vi "Vision Processing.vi"(4 "error in (no error)":errorcluster, 7 "Image Size":T3=enum."320x240") -> ()   [LabVIEW 2016]
doc: "This VI runs in parallel to other tasks. It gets images from the camera, processes them for color or shape and use that information to affect robot behavior."
uses:
  <vilib>/Rock Robotics/WPI/Camera/WPI_CameraImageSize.ctl
  <vilib>/Rock Robotics/WPI/Camera/WPI_CameraWhite Balance Values.ctl
  <vilib>/Rock Robotics/WPI/Camera/WPI_CameraExposure Values.ctl
  <vilib>/Rock Robotics/WPI/Camera/WPI_CameraFrameRate.ctl
  Robot Global Data.vi
panel:
  out "Target Data":T1
  out "Delay":u32
  out "Tiltedness":dbl
  out "Camera Image":T2(plugin-control)
  in  "Vision Target":enum16{"Pegs", "Gears"}(ring)
  out "Binary Image":T2(plugin-control)
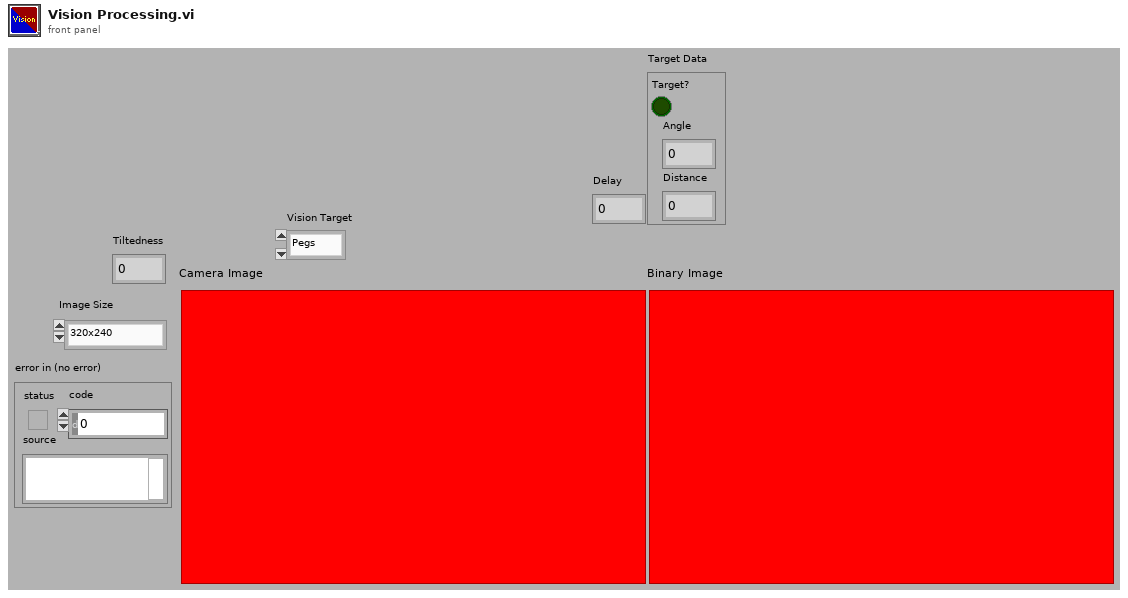
[diagram p1: front panel]
types:
  T1 = cluster{"Target?":bool, "Angle":dbl, "Distance":dbl}
  T2 = typedef "IMAQ Image.ctl" = refnum<image>
  T3 = typedef "WPI_CameraImageSize.ctl" = enum16{"640x480", "320x240", "160x120", "Custom"}
  T4 = typedef "WPI_CameraFrameRate.ctl" = u32
  T5 = typedef "WPI_CameraExposure Values.ctl" = enum16{"Auto", "Flicker-free 50 Hz", "Flicker-free 60 Hz", "Hold current", "Custom"}
  T6 = typedef "WPI_CameraWhite Balance Values.ctl" = enum16{"Auto", "Fixed indoor", "Fixed outdoor 1", "Fixed outdoor 2", "Fixed fluorescent 1", "Fixed fluorescent 2", "Hold current", "Custom"}
  T7 = typedef "Image Type" = u32
  T8 = typedef "WPI_CameraDevRef.ctl" = cluster{"Camera Address":string, "CameraStatus":errorcluster}
  T9 = cluster{"Target?":bool, "PegAngle":dbl, "Distance":dbl}
  T10 = typedef "WPI_EncoderDevRef.ctl" = cluster{"DevStatus":errorcluster, "EncoderIndex":T11, "CounterIndex":T12, "DistancePerCount":dbl, "Decoding Type":T13}
  T11 = typedef "FPGA_EncoderIdx.ctl" = enum8{"Enc 0", "Enc 1", "Enc 2", "Enc 3", "Enc 4", "Enc 5", "Enc 6", "Enc 7", "Invalid"}
  T12 = typedef "FPGA_CounterCtrSystemIndex.ctl" = enum8{"Ctr 0", "Ctr 1", "Ctr 2", "Ctr 3", "Ctr 4", "Ctr 5", "Ctr 6", "Ctr 7", "Invalid"}
  T13 = typedef "WPI_EncoderType.ctl" = enum16{"1x", "2x", "4x"}
  T14 = cluster{"Left":cluster{"L":dbl, "T":dbl, "R":dbl, "B":dbl, "X":dbl, "Y":dbl}, "Right":cluster{"L":dbl, "T":dbl, "R":dbl, "B":dbl, "X":dbl, "Y":dbl}}
  T15 = cluster{"Rectangle":cluster{"L":dbl, "T":dbl, "R":dbl, "B":dbl}, "Center":cluster{"X":dbl, "Y":dbl}}
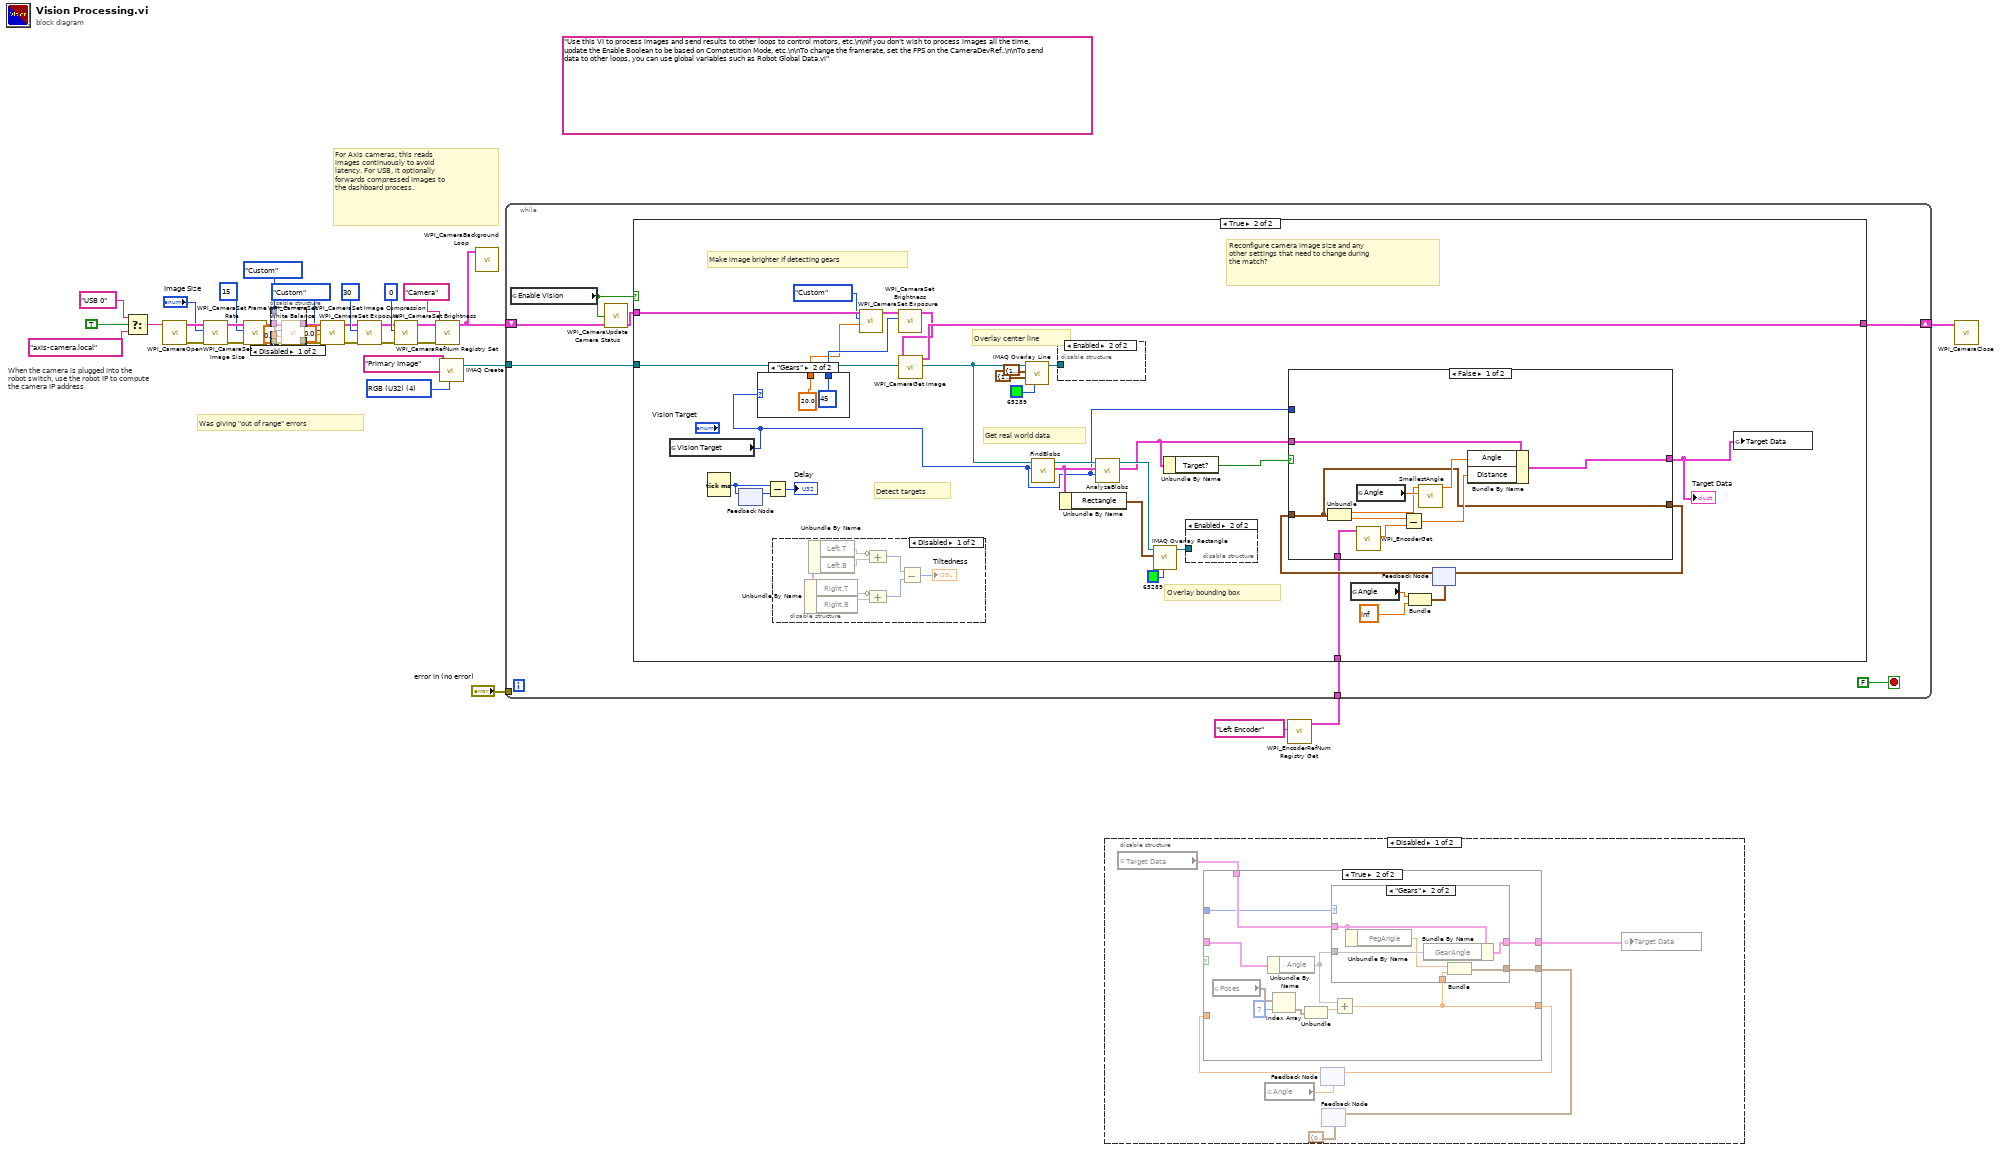
[diagram p0: block diagram]
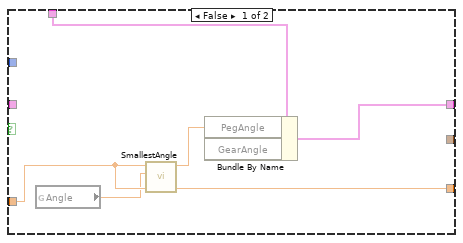
[diagram p2: hidden frame]
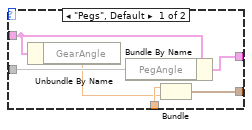
[diagram p3: hidden frame]
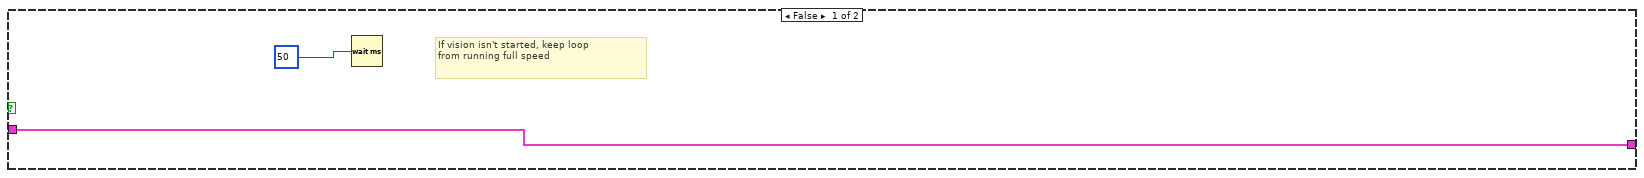
[diagram p6: hidden frame]
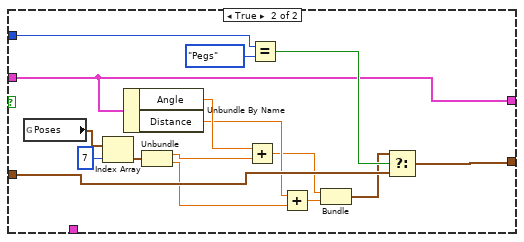
[diagram p7: hidden frame]
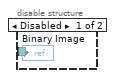
[diagram p9: hidden frame]
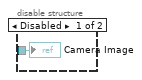
[diagram p10: hidden frame]
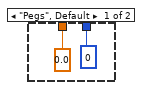
[diagram p11: hidden frame]
diagram:
  (unwired) "Use this VI to process images and send results to other loops to control motors, etc.\n\nIf you don't wish to process images all the time, update the Enable Boolean to be based on Comptetition Mode, etc.\n\nTo change the framerate, set the FPS on the CameraDevRef..\n\nTo send data to other loops, you can use global variables such as Robot Global Data.vi"
  w35 = T7 4 items=["Grayscale (U8)", "Grayscale (I16)", "Grayscale (SGL)", "Complex (CSG)", "RGB (U32)", "HSL (U32)", "RGB (U64)"] ("Image Type")
  # "Was giving \"out of range\" errors"
  # "When the camera is plugged into the\nrobot switch, use the robot IP to compute\nthe camera IP address"
  # "For Axis cameras, this reads\nimages continuously to avoid\nlatency. For USB, it optionally\nforwards compressed images to\nthe dashboard process."
  n1 = Select(t="USB 0" ("format string"), s=TRUE ("dot notation? (F)"), f="axis-camera.local" ("format string")) -> (s? t:f=w6:string)
  n2 = call <vilib>:"WPI_CameraOpen.vi"("Camera Address"=w6) -> ("error out"=w23:errorcluster, "CameraDevRef"=w24:T8)  [unwired: 1 in, 8 out]
  n3 = call <vilib>:"WPI_CameraSet Image Size.vi"("error in (no error)"=w23, "Image Size"="Image Size", "CameraDevRef"=w24) -> ("error out"=w22:errorcluster, "CameraDevRef Out"=w25:T8)  [unwired: 1 in, 6 out]
  n4 = call <vilib>:"WPI_CameraSet Frame Rate.vi"("error in (no error)"=w22, "Frame Rate (fps)"=T4 15, "CameraDevRef"=w25) -> ("error out"=w21:errorcluster, "CameraDevRef Out"=w27:T8)  [unwired: 7 out]
  n5 = disable-structure shown="Disabled" {
    disable-tunnel: w27 -> [w41 w43]
    disable-tunnel: [w40 w43] -> w26
    disable-tunnel: w21 -> [w39 w42]
    disable-tunnel: [w38 w42] -> w20
    disable-tunnel: WPI_CameraWhite_Balance_Values."Custom" ("White Balance") -> [w37 _]
    disable-tunnel: 0.0 ("Color Temp (K)") -> [w36 _]
    frame Disabled {
      n6 = call <vilib>:"WPI_CameraSet White Balance.vi"("error in (no error)"=w39, "Color Temp (K)"=w36, "White Balance"=w37, "CameraDevRef"=w41) -> ("error out"=w38:errorcluster, "CameraDevRef Out"=w40:T8)  [unwired: 6 out]
    }
    frame Enabled {
    }
  }
  n7 = call <vilib>:"WPI_CameraSet Exposure.vi"("error in (no error)"=w20, "Exposure (%)"=0.0, "Exposure"=WPI_CameraExposure_Values."Custom", "CameraDevRef"=w26) -> ("error out"=w19:errorcluster, "CameraDevRef Out"=w29:T8)  [unwired: 6 out]
  n8 = call <vilib>:"WPI_CameraSet Image Compression.vi"("error in (no error)"=w19, "Compression"=30, "CameraDevRef"=w29) -> ("error out"=w18:errorcluster, "CameraDevRef Out"=w28:T8)  [unwired: 7 out]
  n9 = call <vilib>:"WPI_CameraSet Brightness.vi"("error in (no error)"=w18, "Brightness"=0, "CameraDevRef"=w28) -> ("error out"=w16:errorcluster, "CameraDevRef Out"=w17:T8)  [unwired: 7 out]
  n10 = call <vilib>:"WPI_CameraRefNum Registry Set.vi"("error in (no error)"=w16, "refnum name"="Camera", "CameraDevRef"=w17) -> ("CameraDevRef"=w12:T8)  [unwired: 1 in, 7 out]
  n11 = call "IMAQ Create"("Image Name"="Primary Image", "Image Type"=w35) -> ("New Image"=w33:T2)  [unwired: 2 in, 2 out]
  n12 = call <vilib>:"WPI_CameraBackground Loop.vi"("CameraDevRef"=w12) -> ()  [unwired: 11 in]
  n13 = disable-structure shown="Disabled" {
    frame Disabled {
      n14 = global read "Robot Global Data.vi" "Target Data"() -> (w47:T9)
      n15 = global read "Robot Global Data.vi" "Angle"() -> (w48:dbl)
      n16 = feedback #1(w48) -> (w50:dbl)
      n17 = case shown="True" {
        selector: _ -> [_ _]
        tunnel: [w55 w59] -> w46
        tunnel: _ -> [_ w60]
        tunnel: [w54 w56] -> w49
        tunnel: w50 -> [w54 _]
        tunnel: w47 -> [w51 w62]
        tunnel: _ -> [_ w58]
        tunnel: [_ w57] -> w44
        frame False {
          n18 = global read "Robot Global Data.vi" "Angle"() -> (w53:dbl)
          n19 = call "SmallestAngle.vi"("Angle 2"=w53, "Angle 1"=w54) -> ("Smallest Difference"=w52:dbl)  [unwired: 9 in]
          n20 = Bundle By Name(cluster=w51, "PegAngle"=w52) -> (w55:T9)  [unwired: 1 in]
        }
        frame True {
          n21 = global read "Robot Global Data.vi" "Poses"() -> (w66:cluster{"theta":dbl, "distance":dbl}[])
          n22 = Unbundle By Name(w60) -> ("Angle"=w61)
          n23 = Index Array(array=w66, index=7) -> (element=w64:cluster{"theta":dbl, "distance":dbl})
          n24 = Unbundle(w64) -> ("theta"=w63:dbl)  [unwired: 1 out]
          n25 = Add(x=w61, y=w63) -> (x+y=w56:dbl)
          n26 = case shown="\"Gears\"" w58 {
            tunnel: w62 -> [w68 w74]
            tunnel: w61 -> [w71 w78]
            tunnel: [w72 w77] -> w59
            tunnel: [w70 w75] -> w57
            tunnel: w56 -> [w69 w76]
            frame "Pegs", Default {
              n27 = Unbundle By Name(w68) -> ("GearAngle"=w67:dbl)
              n28 = Bundle By Name(cluster=w68, "PegAngle"=w71) -> (w72:T9)
              n29 = Bundle(w69, "GearAngle"=w67) -> (w70:cluster{dbl, "GearAngle":dbl})  [unwired: 1 in]
            }
            frame "Gears" {
              n30 = Unbundle By Name(w74) -> ("PegAngle"=w73:dbl)
              n31 = Bundle By Name(cluster=w74, "GearAngle"=w78) -> (w77:T9)
              n32 = Bundle("PegAngle"=w73, w76) -> (w75:cluster{"PegAngle":dbl, dbl})  [unwired: 1 in]
            }
          }
        }
      }
      n33 = feedback-in #1(w49) -> ()
      n34 = feedback #2(cluster{"PegAngle":dbl, "GearAngle":dbl} {"PegAngle"=0.0, "GearAngle"=0.0} ("Target Data")) -> ()  [unwired: 1 in]
      n35 = feedback-in #2(w44) -> ()
      n36 = global write "Robot Global Data.vi" "Target Data"(w46) -> ()
    }
    frame Enabled {
    }
  }
  n37 = call <vilib>:"WPI_EncoderRefNum Registry Get.vi"("refnum name"="Left Encoder") -> ("EncoderDevRef"=w1:T10)  [unwired: 9 in, 1 out]
  n38 = while {
    shift-right: [w84] -> w10
    shift-left: w12 -> [w82]
    tunnel: w33 -> [w83]
    tunnel: "error in (no error)" -> [_]
    tunnel: w1 -> [w79]
    stop <- FALSE stop-if-true
    n39 = global read "Robot Global Data.vi" "Enable Vision"() -> (w80:bool)
    n40 = call <vilib>:"WPI_CameraUpdate Camera Status.vi"("CameraDevRef In"=w82, "Enable Vision"=w80) -> ("CameraDevRef Out"=w81:T8)  [unwired: 3 in]
    n41 = case shown="True" w80 {
      tunnel: w83 -> [_ w119]
      tunnel: [w87 w118] -> w84
      tunnel: w81 -> [w87 w107]
      tunnel: w79 -> [_ w91]
      frame False {
        # "If vision isn't started, keep loop\nfrom running full speed"
        n42 = Wait (ms)(milliseconds to wait=u32 50) -> ()  [unwired: 1 out]
      }
      frame True {
        # "Get real world data"
        # "Detect targets"
        # "Make image brighter if detecting gears"
        # "Overlay center line"
        # "Overlay bounding box"
        # "Reconfigure camera image size and any\nother settings that need to change during\nthe match?"
        n43 = global read "Robot Global Data.vi" "Vision Target"() -> (w93:enum16{"Pegs", "Gears"})
        n44 = Tick Count (ms)() -> (millisecond timer value=w102:u32)
        n45 = feedback-in #3(w102) -> ()
        n46 = feedback #3() -> (w103:u32)  [unwired: 1 in]
        n47 = case shown="\"Gears\"" w93 {
          tunnel: [0 ("Brightness") 45 ("Brightness")] -> w105
          tunnel: [0.0 ("Color Temp (K)") 20.0 ("Color Temp (K)")] -> w104
          frame "Pegs", Default {
          }
          frame "Gears" {
          }
        }
        n48 = Subtract(x=w102, y=w103) -> (x-y=→"Delay":u32)
        n49 = disable-structure shown="Disabled" {
          frame Disabled {
            n50 = Unbundle By Name() -> (w153:T14, "Left.T"=w152, "Left.B"=w151)
            n51 = Unbundle By Name(w153) -> ("Right.T"=w150, "Right.B"=w149)
            n52 = Compound Arithmetic op=ADD(invert w152, w151) -> (w148:i32)
            n53 = Compound Arithmetic op=ADD(invert w150, w149) -> (w147:i32)
            n54 = Subtract(x=w148, y=w147) -> (x-y=→"Tiltedness":i32)
          }
          frame Enabled {
          }
        }
        n55 = call <vilib>:"WPI_CameraSet Exposure.vi"("Exposure (%)"=w104, "Exposure"=WPI_CameraExposure_Values."Custom", "CameraDevRef"=w107) -> ("CameraDevRef Out"=w100:T8)  [unwired: 1 in, 7 out]
        n56 = call <vilib>:"WPI_CameraSet Brightness.vi"("Brightness"=w105, "CameraDevRef"=w100) -> ("CameraDevRef Out"=w106:T8)  [unwired: 1 in, 8 out]
        n57 = call <vilib>:"WPI_CameraGet Image.vi"("Image"=w119, "CameraDevRef"=w106) -> ("Image Out"=w109:T2, "CameraDevRef Out"=w118:T8)  [unwired: 1 in, 7 out]
        n58 = call "IMAQ Overlay Line"("Color"=u32 65289, "End Point"=cluster{"X":i32, "Y":i32} {"X"=160, "Y"=240}, "Start Point"=cluster{"X":i32, "Y":i32} {"X"=160, "Y"=0}, "Image"=w109) -> ("Image Out"=w108:T2)  [unwired: 6 in, 1 out]
        n59 = call "FindBlobs.vi"("Vision Target"=w93, "Image In"=w109) -> ("Blob Data"=w114:T15, "Image Out"=w98:T2)  [unwired: 8 in]
        n60 = disable-structure shown="Enabled" {
          disable-tunnel: w108 -> [w155 _]
          frame Disabled {
            "Camera Image" <- w155
          }
          frame Enabled {
          }
        }
        n61 = Unbundle By Name(w114) -> ("Rectangle"=w113:cluster{"L":dbl, "T":dbl, "R":dbl, "B":dbl})
        n62 = call "AnalyzeBlobs.vi"("Vision Target"=w93, "Blob Data"=w114, "Image In"=w98) -> ("Target Data"=w96:T1, "Image Out"=w115:T2)  [unwired: 7 in]
        n63 = call "IMAQ Overlay Rectangle"("Color"=u32 65289, "Rectangle"=w113, "Image"=w115) -> ("Image Out"=w116:T2)  [unwired: 7 in, 1 out]
        n64 = Unbundle By Name(w96) -> ("Target?"=w97:bool)
        n65 = disable-structure shown="Enabled" {
          disable-tunnel: w116 -> [w154 _]
          frame Disabled {
            "Binary Image" <- w154
          }
          frame Enabled {
          }
        }
        n66 = global read "Robot Global Data.vi" "Angle"() -> (w90:dbl)
        n67 = Bundle("Angle"=w90, "Distance"=inf) -> (w89:cluster{"Angle":dbl, "Distance":dbl})  [unwired: 1 in]
        n68 = feedback #4(w89) -> (w95:cluster{"Angle":dbl, "Distance":dbl})
        n69 = case shown="False" w97 {
          tunnel: w96 -> [w127 w138]
          tunnel: [w120 w133] -> w94
          tunnel: w95 -> [w120 w139]
          tunnel: w93 -> [_ w142]
          tunnel: [w126 w138] -> w92
          tunnel: w91 -> [w124 _]
          frame False {
            n70 = Unbundle(w120) -> ("Angle"=w125:dbl, "Distance"=w123:dbl)
            n71 = global read "Robot Global Data.vi" "Angle"() -> (w129:dbl)
            n72 = call <vilib>:"WPI_EncoderGet.vi"("EncoderDevRef"=w124) -> ("Distance"=w122:dbl)  [unwired: 5 in, 5 out]
            n73 = Subtract(x=w123, y=w122) -> (x-y=w121:dbl)
            n74 = call "SmallestAngle.vi"("Angle 2"=w129, "Angle 1"=w125) -> ("Smallest Difference"=w128:dbl)  [unwired: 9 in]
            n75 = Bundle By Name(cluster=w127, "Angle"=w128, "Distance"=w121) -> (w126:T1)
          }
          frame True {
            n76 = global read "Robot Global Data.vi" "Poses"() -> (w145:cluster{"theta":dbl, "distance":dbl}[])
            n77 = Index Array(array=w145, index=7) -> (element=w132:cluster{"theta":dbl, "distance":dbl})
            n78 = Unbundle By Name(w138) -> ("Angle"=w143:dbl, "Distance"=w137:dbl)
            n79 = Unbundle(w132) -> ("theta"=w131:dbl, "distance"=w130:dbl)
            n80 = Add(x=w143, y=w131) -> (x+y=w135:dbl)
            n81 = Equal?(x=w142, y=enum16{"Pegs", "Gears"}."Pegs") -> (x = y?=w140:bool)
            n82 = Add(x=w137, y=w130) -> (x+y=w136:dbl)
            n83 = Bundle(w135, w136) -> (w134:cluster{dbl, dbl})  [unwired: 1 in]
            n84 = Select(t=w134, s=w140, f=w139) -> (s? t:f=w133:cluster{"Angle":dbl, "Distance":dbl})
          }
        }
        "Target Data" <- w92
        n85 = feedback-in #4(w94) -> ()
        n86 = global write "Robot Global Data.vi" "Target Data"(w92) -> ()
      }
    }
  }
  n87 = call <vilib>:"WPI_CameraClose.vi"("CameraDevRef"=w10) -> ()  [unwired: 1 in, 10 out]
